vi "Fourth Ex.vi"() -> ()   [LabVIEW 2016]
panel:
  out "# of Loops":i32
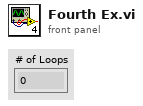
[diagram p1: front panel]
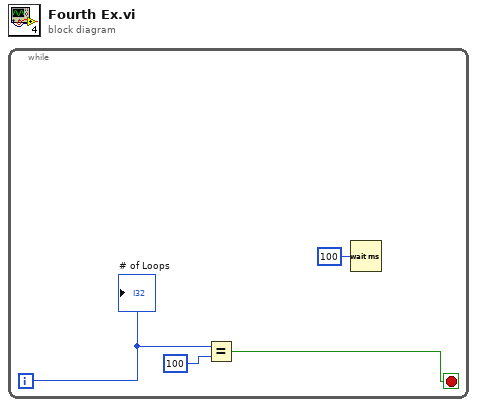
[diagram p0: block diagram]
diagram:
  n1 = while {
    i -> [w4]
    stop <- w2 stop-if-true
    n2 = Equal?(x=w4, y=100) -> (x = y?=w2:bool)
    n3 = Wait (ms)(milliseconds to wait=u32 100) -> ()  [unwired: 1 out]
    "# of Loops" <- w4
  }
